vi "refresh user interface.vi"(8 "channel names (combo box labels)":string[](array[string]), 9 "combo box references":refnum<vi>[](array[refnum]), 10 "engine configuration":refnum<class "engine configuration.lvclass">, 11 "control module configuration in":refnum<class "control module configuration.lvclass">) -> ()   [LabVIEW 2013, in "My Awesome Control Modules editor node.lvclass"]
uses:
  My Awesome Control Modules editor node.lvclass
  <vilib>/NI/Tag Bus Data Framework/control module/configuration/control module configuration.lvclass
  <vilib>/NI/Tag Bus/tag/tag descriptor.lvclass
  <vilib>/NI/Module Execution Interface/Engine Configuration/engine configuration.lvclass
  <vilib>/NI/Configuration Framework/serializable configuration/NISE_CEF_serializable configuration.lvclass
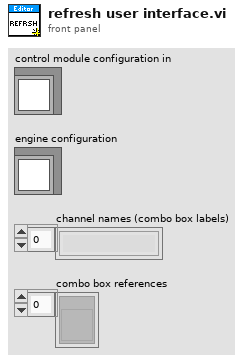
[diagram p1: front panel]
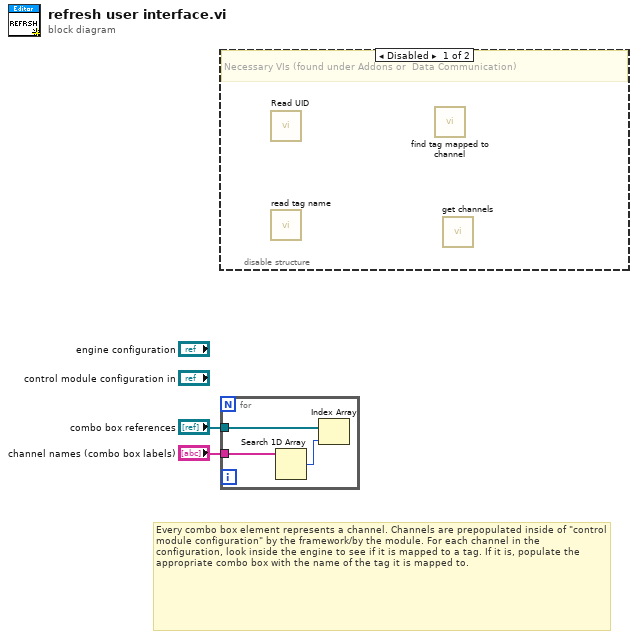
[diagram p0: block diagram]
diagram:
  # "Every combo box element represents a channel. Channels are prepopulated inside of \"control module configuration\" by the framework/by the module. For each channel in the configuration, look inside the engine to see if it is mapped to a tag. If it is, populate the appropriate combo box with the name of the tag it is mapped to."
  n1 = disable-structure shown="Disabled" {
    frame Disabled {
      # "Necessary VIs (found under Addons or  Data Communication)"
      n2 = call <vilib>:"Read UID.vi"() -> ()  [unwired: 9 in, 3 out]
      n3 = call <vilib>:"read tag name.vi"() -> ()  [unwired: 9 in, 3 out]
      n4 = call <vilib>:"find tag mapped to channel.vi"() -> ()  [unwired: 9 in, 3 out]
      n5 = call-dynamic "get channels.vi"() -> ()  [unwired: 10 in, 2 out]
    }
    frame Enabled {
    }
  }
  n6 = for {
    tunnel: "channel names (combo box labels)" -> [w5]
    tunnel: "combo box references" -> [w3]
    n7 = Search 1D Array(1D array=w5) -> (index of element=w4:i32)  [unwired: 2 in]
    n8 = Index Array(array=w3, index=w4) -> ()  [unwired: 1 out]
  }
